vi "Start.vi"(8 "error in (no error)":errorcluster, 11 "Task in":refnum<class "DSP.lvclass">) -> (0 "error out":errorcluster, 3 "Task out":refnum<class "DSP.lvclass">)   [LabVIEW 2009, in "MicroDAQ.lvlib" / "DSP.lvclass"]
uses:
  <instrlib>/MicroDAQ/Channel/DSP/DSP.lvclass
  <instrlib>/MicroDAQ/Mlink library wraper/mlink.lvlib
  <instrlib>/MicroDAQ/Channel/Channel.lvclass
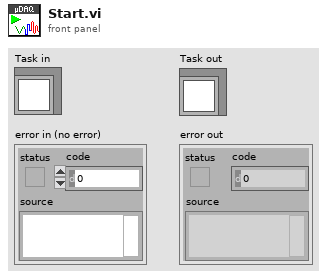
[diagram p1: front panel]
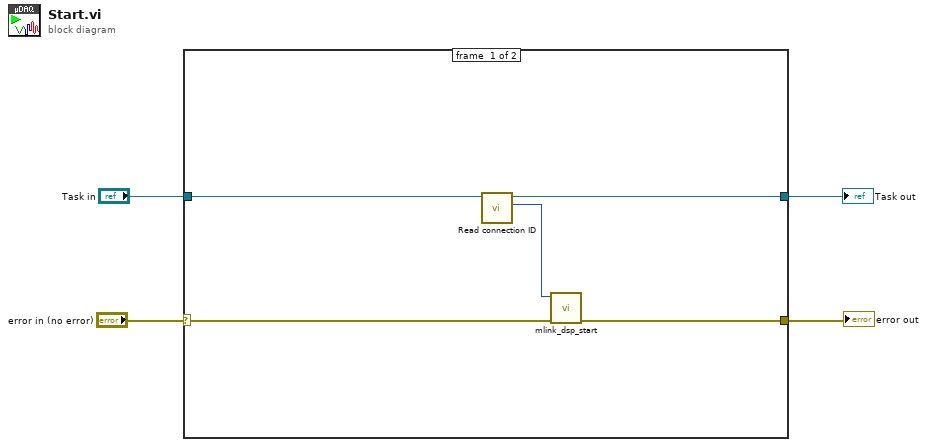
[diagram p0: block diagram]
diagram:
  n1 = case shown="No Error" "error in (no error)" {
    selector: "error in (no error)" -> [w6 w11]
    tunnel: [w5 w11] -> w3
    tunnel: "Task in" -> [w9 w10]
    tunnel: [w8 w10] -> w1
    frame #0 {
      n2 = call <instrlib>:"Read connection ID.vi"("Task in"=w9) -> ("connection ID"=w7:i32, "Task out"=w8:refnum<class "DSP.lvclass">)  [unwired: 9 in]
      n3 = call <instrlib>:"mlink_dsp_start.vi"("error in (no error)"=w6, "connection ID"=w7) -> ("error out"=w5:errorcluster)  [unwired: 8 in, 1 out]
    }
    frame #1 {
    }
  }
  "error out" <- w3
  "Task out" <- w1
